vi "AI 5783.vi"() -> (4 "i18x1":fxp<+/-,18,1>[](array[numeric]) format="%.18g", 10 "output valids":bool[](array[boolean]))   [LabVIEW 2017, in "Lock-In Amplifier Example FPGA.lvlib"]
uses:
  Lock-In Amplifier Example FPGA.lvlib
  <vilib>/eio/EIONode/EIONode.xnode
  <vilib>/rvi/eio/common/nirviEmuTemplateMethod_errors.vi
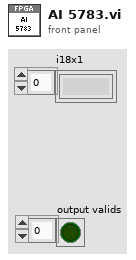
[diagram p1: front panel]
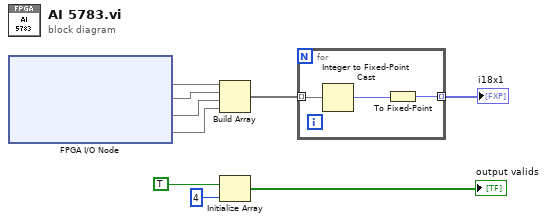
[diagram p0: block diagram]
diagram:
  n1 = xnode "FPGA I/O Node"() -> ("IO Module\\AI 0 Data N"=w9, "IO Module\\AI 1 Data N"=w8, "IO Module\\AI 2 Data N"=w7, "IO Module\\AI 3 Data N"=w6)  [unwired: 4 in, 4 out]
  n2 = Build Array(w9, w8, w7, w6) -> (w2:void[])
  n3 = Initialize Array(TRUE, 4 ("dimension size")) -> (→"output valids":bool[])
  n4 = for {
    tunnel: w2 -> [w11] mode=indexing
    tunnel: [w10] -> w1 mode=indexing
    n5 = Integer to Fixed-Point Cast(integer=w11) -> (fixed-point=w12:fxp<+/-,16,1>)  [unwired: 1 in]
    n6 = To Fixed-Point(number=w12) -> (fixed-point=w10:fxp<+/-,18,1>)  [unwired: 1 in]
  }
  "i18x1" <- w1
